vi "GraphView(Cursor).vi"() -> ()   [LabVIEW 2014]
uses:
  <vilib>/Utility/miscctls.llb/LVCursorListTypeDef.ctl
  GlobalData/GlobalData.vi
panel:
  out "クラスタ 2":T1
  out "クラスタ":T1
  in  "中央に表示A":bool
  in  "対象スケール(Y)":u16(ring) items=["回転M1１", "回転M23", "トルクM1", "トルクM23", "温度１", "温度２", "温度３", "温度４"]
  in  "削除B":bool
  in  "カーソル名称":string
  in  "カーソルB":u16(ring) items=["あ", "い"]
  in  "カーソルA":u16(ring) items=["あ", "い"]
  in  "トレース追加ボタン":bool
  in  "削除A":bool
  in  "表 2":string[][](table)
  in  "カラー":u32(colorbox)
  in  "カーソルモード":u16(ring) items=["フリー", "データ"]
  in  "対象CH":u16(ring) items=["自動", "No.", "時間HH:MM:SS.S", "M1回転rpm", "M2回転rpm", "M3回転rpm", "M1トルクN･m", "M2トルクN･m", "M3トルクN･m", "", "", "", "", "", "", "", "", "", "", "供試体温度1℃", "供試体温度2℃", "供試体温度3℃", "動力盤温度℃", "軸受温度1℃", "軸受温度2℃", "軸受温度3℃", "", "効率"]
  out "カーソルリスト":T2
  out "表":string[][](table)
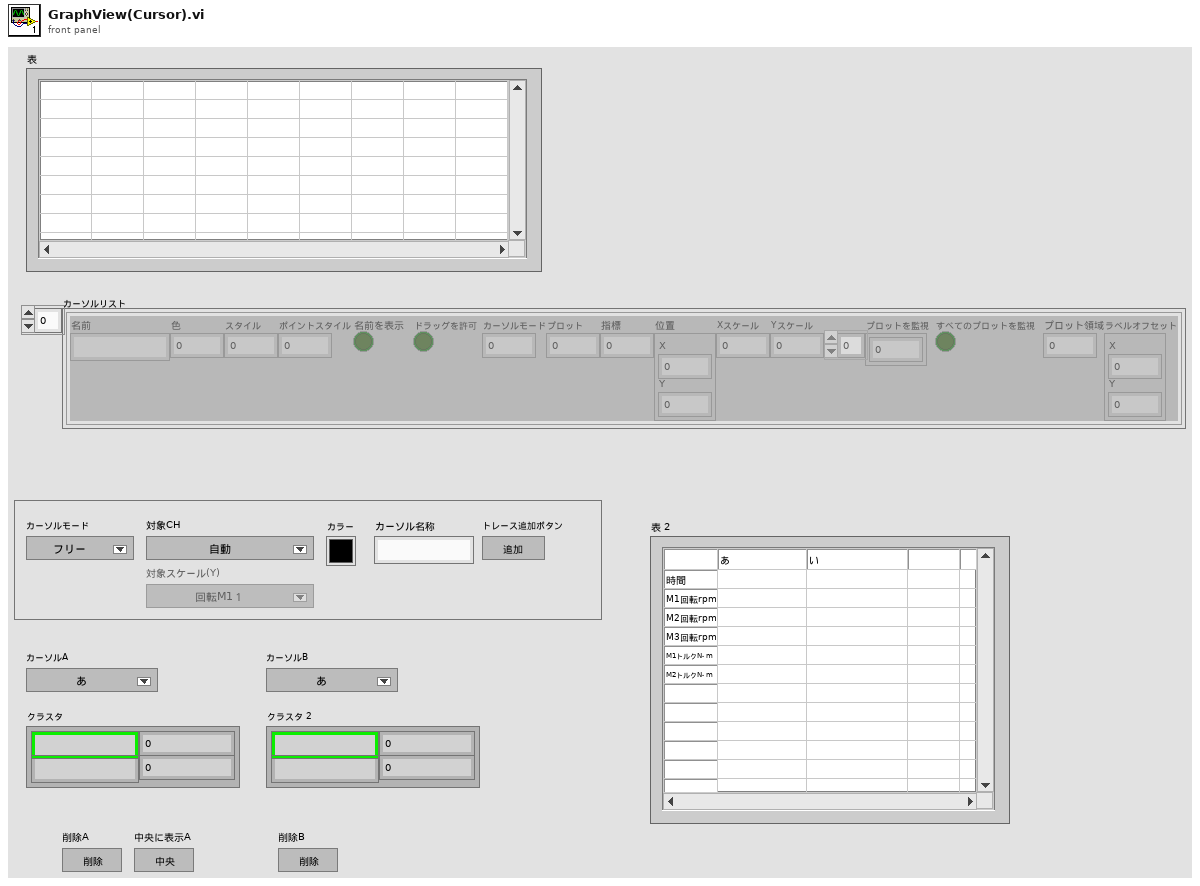
[diagram p1: front panel]
types:
  T1 = cluster{"X軸名":string, "X値":dbl, "Y軸名":string, "Y値":dbl}
  T2 = typedef "LVCursorListTypeDef.ctl" = cluster{"Name":string, "Color":u32, "Style":u8, "Point Style":u8, "Name Visible":bool, "Allow Drag":bool, "Cursor Mode":u32, "Plot":i32, "Index":i32, "Position":cluster{"X":dbl, "Y":dbl}, "X Scale":u32, "Y Scale":u32, "Watch Plots":i32[], "Watch All Plots":bool, "Plot Area":i32, "Label Offset":cluster{"X":dbl, "Y":dbl}}[]
  T3 = enum8{"Enabled", "Disabled", "Disabled and Grayed Out"}
  T4 = cluster{"Name":string, "Color":u32, "Style":u8, "Point Style":u8, "Name Visible":bool, "Allow Drag":bool, "Cursor Mode":u32, "Plot":i32, "Index":i32, "Position":cluster{"X":dbl, "Y":dbl}, "X Scale":u32, "Y Scale":u32, "Watch Plots":i32[], "Watch All Plots":bool, "Plot Area":i32, "Label Offset":cluster{"X":dbl, "Y":dbl}}
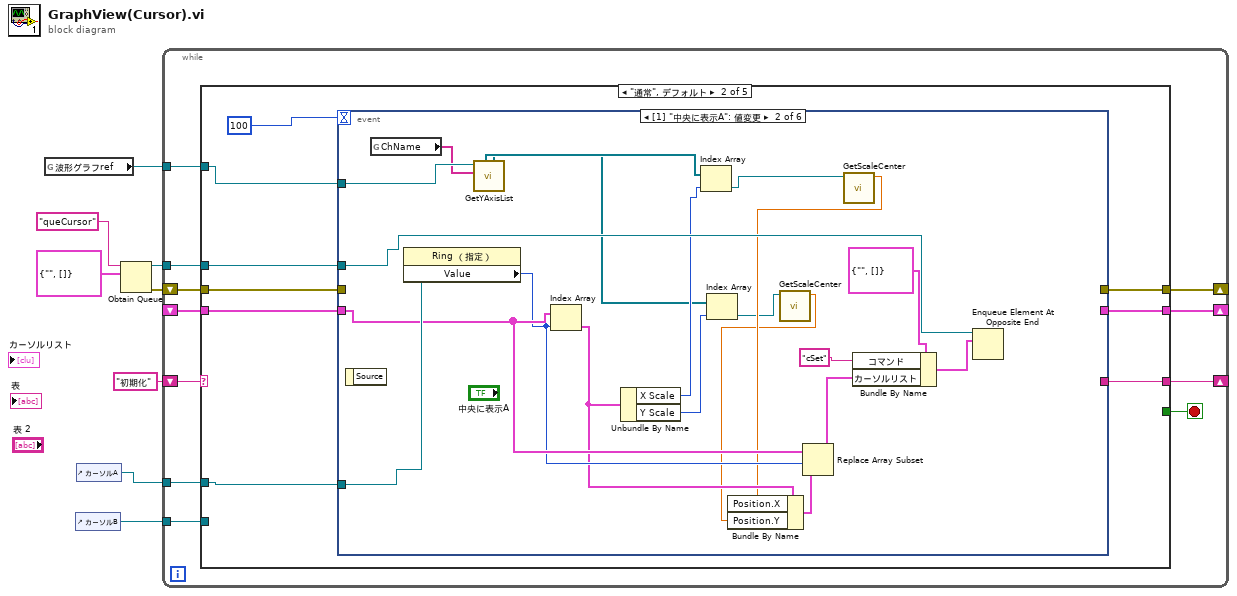
[diagram p0: block diagram]
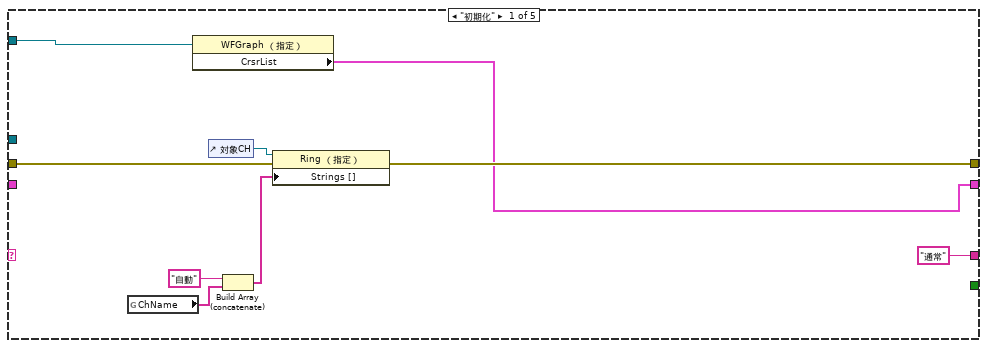
[diagram p2: hidden frame]
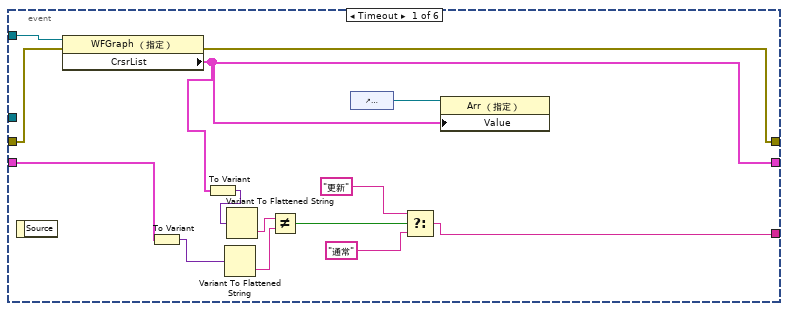
[diagram p3: hidden frame]
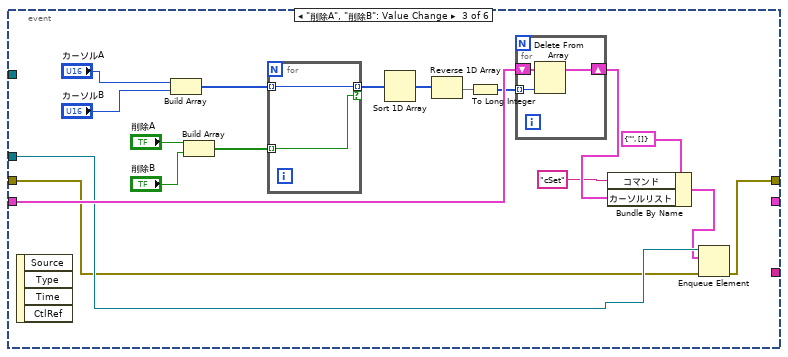
[diagram p4: hidden frame]
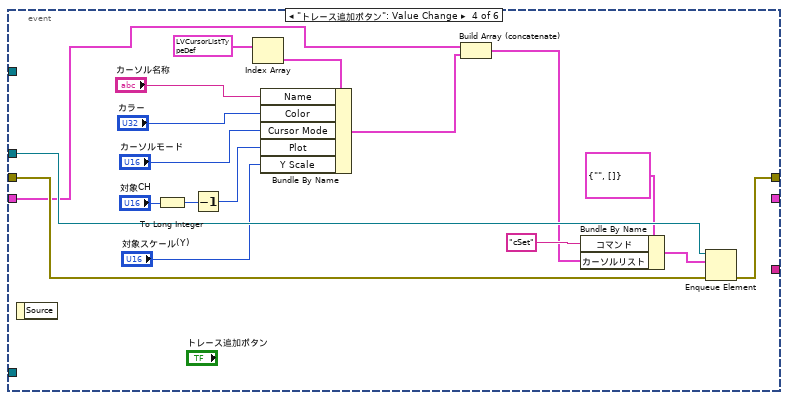
[diagram p5: hidden frame]
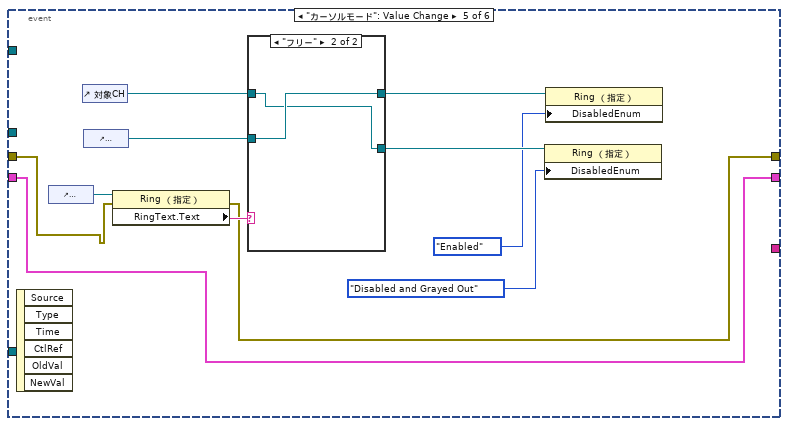
[diagram p6: hidden frame]
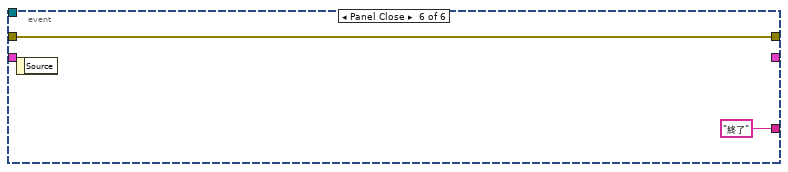
[diagram p8: hidden frame]
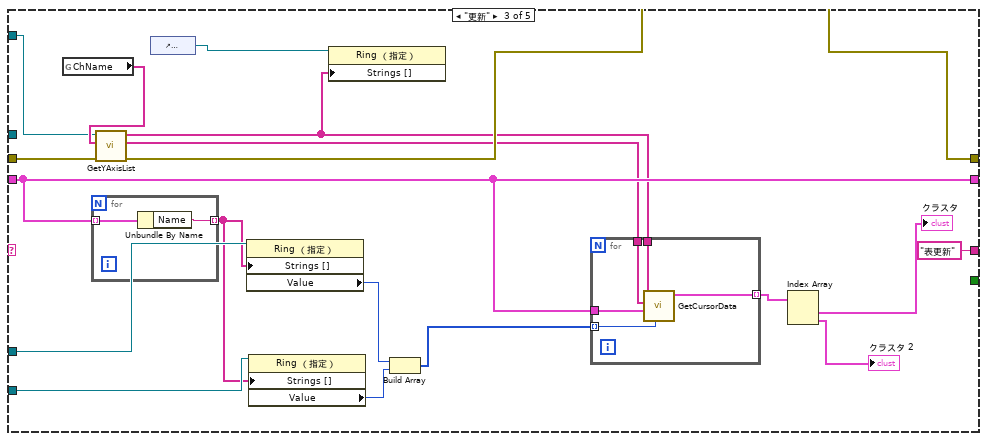
[diagram p9: hidden frame]
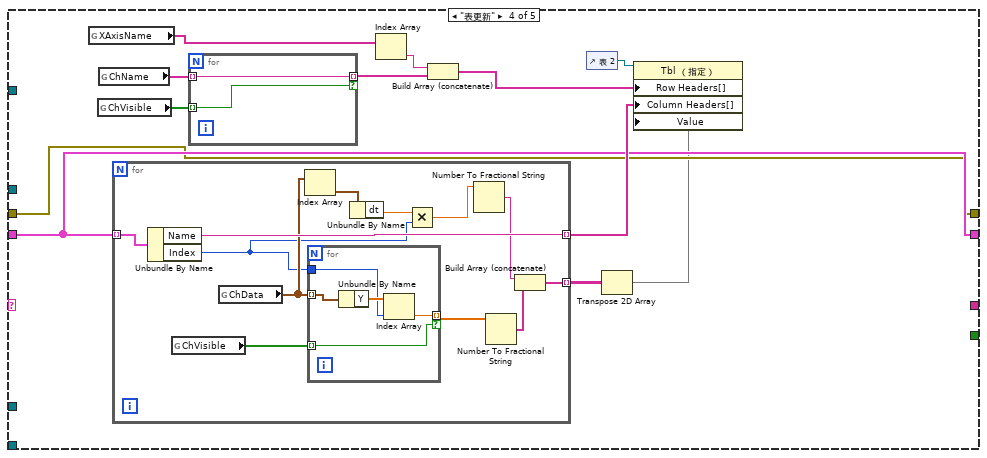
[diagram p10: hidden frame]
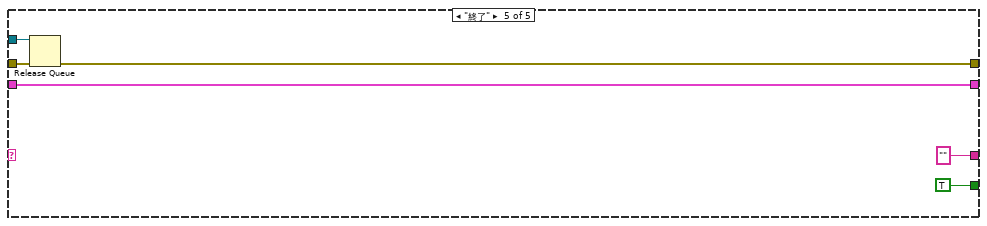
[diagram p11: hidden frame]
diagram:
  n1 = global read "GlobalData.vi" "波形グラフref"() -> (w3:refnum<vi>)
  n2 = control-ref of="カーソルB"() -> (w1:refnum<vi>)
  n3 = control-ref of="カーソルA"() -> (w2:refnum<vi>)
  n4 = Obtain Queue(name (unnamed)="queCursor" ("名前（名前なし）"), element data type=cluster{"コマンド":string, "カーソルリスト":T2} {"コマンド"="", "カーソルリスト"=[]}) -> (queue out=w4:refnum<queue>, error out=w7:errorcluster)  [unwired: 3 in, 1 out]
  n5 = while {
    tunnel: w4 -> [w17]
    shift-right: [w16] -> _
    shift-left: w7 -> [w18]
    shift-right: [w14] -> _
    shift-left: "初期化" -> [w15]
    shift-right: [w13] -> _
    shift-left: _ -> [w12]
    tunnel: w3 -> [w11]
    tunnel: w2 -> [w10]
    tunnel: w1 -> [w9]
    stop <- w19 stop-if-true
    n6 = case shown="\"通常\", デフォルト" w15 {
      tunnel: [_ _ _ _ TRUE] -> w19
      tunnel: w18 -> [w27 w37 w145 w156 w189]
      tunnel: w17 -> [_ w35 _ _ w187]
      tunnel: [w26 w34 w144 w156 w188] -> w16
      tunnel: ["通常" w33 "表更新" _ ""] -> w14
      tunnel: [w20 w32 w147 w157 w186] -> w13
      tunnel: w12 -> [_ w31 w147 w157 w186]
      tunnel: w11 -> [w21 w30 w139 _ _]
      tunnel: w10 -> [_ w29 w146 _ _]
      tunnel: w9 -> [_ _ w138 _ _]
      frame "初期化" {
        n7 = global read "GlobalData.vi" "ChName"() -> (w23:string[])
        n8 = property class="WFGraph （指定）"(reference=w21) -> ("CrsrList"=w20:T2)  [unwired: 1 in, 2 out]
        n9 = control-ref of="対象CH"() -> (w25:refnum<vi>)
        n10 = Build Array (concatenate)("自動", w23) -> (w22:string[])
        n11 = property class="Ring （指定）"(reference=w25, error in=w27, "Strings []"=w22) -> (error out=w26:errorcluster)  [unwired: 1 out]
      }
      frame "通常", Default {
        n12 = event shown="[1] \"中央に表示A\": 値変更" {
          selector: _ -> [_ _ _ _ _ _]
          dyn-events: _ -> [_ _ _ _ _ _]
          timeout: 100 -> [_ _ _ _ _ _]
          tunnel: w37 -> [w49 _ w73 w108 w115 w129]
          tunnel: w35 -> [_ w70 w78 w112 _ _]
          tunnel: [w48 _ w72 w107 w114 w129] -> w34
          tunnel: [w38 _ _ _ _ "終了"] -> w33
          tunnel: [w42 _ _ _ w113 _] -> w32
          tunnel: w31 -> [w46 w60 w81 w97 w113 _]
          tunnel: w30 -> [w50 w67 _ _ _ _]
          tunnel: w29 -> [_ w71 _ _ _ _]
          event Timeout {
            n13 = event-data() -> ()  [unwired: 1 in, 1 out]
            n14 = property class="WFGraph （指定）"(reference=w50, error in=w49) -> (error out=w48:errorcluster, "CrsrList"=w42:T2)  [unwired: 1 out]
            n15 = To Variant(anything=w46) -> (Variant=w45:variant)
            n16 = To Variant(anything=w42) -> (Variant=w47:variant)
            n17 = Variant To Flattened String(Variant=w45) -> (data string=w43:string)  [unwired: 1 out]
            n18 = Variant To Flattened String(Variant=w47) -> (data string=w44:string)  [unwired: 1 out]
            n19 = Not Equal?(x=w44, y=w43) -> (x != y?=w41:bool)
            n20 = control-ref of="カーソルリスト"() -> (w51:refnum<vi>)
            n21 = Select(t="更新", s=w41, f="通常") -> (s? t:f=w38:string)
            n22 = property class="Arr （指定）"(reference=w51, "Value"=w42) -> ()  [unwired: 1 in, 2 out]
          }
          event "中央に表示A": Value Change {
            n23 = event-data() -> ()  [unwired: 1 in, 1 out]
            n24 = global read "GlobalData.vi" "ChName"() -> (w66:string[])
            n25 = property class="Ring （指定）"(reference=w71) -> ("Value"=w59:u16)  [unwired: 1 in, 2 out]
            n26 = call "GetYAxisList.vi"("ChName[]"=w66, "波形グラフref"=w67) -> ("Y軸ref[]"=w63:refnum<vi>[], "X軸ref[]"=w65:refnum<vi>[])  [unwired: 4 in, 4 out]
            n27 = Index Array(array=w60, index=w59) -> (element=w58:T4)
            n28 = Unbundle By Name(w58) -> ("X Scale"=w64:u32, "Y Scale"=w62:u32)
            n29 = Index Array(array=w65, index=w64) -> (element=w57:refnum<vi>)
            n30 = Index Array(array=w63, index=w62) -> (element=w55:refnum<vi>)
            n31 = call "GetScaleCenter.vi"("GraphScale入力"=w55) -> ("数値"=w54:dbl)  [unwired: 10 in]
            n32 = call "GetScaleCenter.vi"("GraphScale入力"=w57) -> ("数値"=w56:dbl)  [unwired: 10 in]
            n33 = Bundle By Name(cluster=w58, "Position.X"=w56, "Position.Y"=w54) -> (w53:T4)
            n34 = Replace Array Subset(array=w60, new element=w53, index=w59) -> (w61:T2)
            n35 = Bundle By Name(cluster=cluster{"コマンド":string, "カーソルリスト":T2} {"コマンド"="", "カーソルリスト"=[]}, "コマンド"="cSet", "カーソルリスト"=w61) -> (w52:cluster{"コマンド":string, "カーソルリスト":T2})
            n36 = Enqueue Element At Opposite End(queue=w70, element=w52) -> ()  [unwired: 2 in, 3 out]
          }
          event "削除A", "削除B": Value Change {
            n37 = event-data() -> ()  [unwired: 1 in, 4 out]
            n38 = Build Array("カーソルA", "カーソルB") -> (w85:u16[])
            n39 = Build Array("削除A", "削除B") -> (w84:bool[])
            n40 = for {
              tunnel: w85 -> [w94] mode=indexing
              tunnel: w84 -> [w93] mode=indexing
              tunnel: [w94] -> w83 mode=indexing if=w93
            }
            n41 = Sort 1D Array(array=w83) -> (sorted array=w82:u16[])
            n42 = Reverse 1D Array(array=w82) -> (reversed array=w80:u16[])
            n43 = To Long Integer(number=w80) -> (32bit integer=w79:i32[])
            n44 = for {
              tunnel: w79 -> [w91] mode=indexing
              shift-right: [w90] -> w76
              shift-left: w81 -> [w92]
              n45 = Delete From Array(array=w92, index=w91) -> (array with subset deleted=w90:T2)  [unwired: 1 in, 1 out]
            }
            n46 = Bundle By Name(cluster=cluster{"コマンド":string, "カーソルリスト":T2} {"コマンド"="", "カーソルリスト"=[]} ("要素"), "コマンド"="cSet", "カーソルリスト"=w76) -> (w74:cluster{"コマンド":string, "カーソルリスト":T2})
            n47 = Enqueue Element(queue=w78, element=w74, error in (no error)=w73) -> (error out=w72:errorcluster)  [unwired: 1 in, 2 out]
          }
          event "トレース追加ボタン": Value Change {
            n48 = event-data() -> ()  [unwired: 1 in, 1 out]
            n49 = To Long Integer(number="対象CH") -> (32bit integer=w99:i32)
            n50 = Decrement(x=w99) -> (x-1=w98:i32)
            n51 = Index Array(array=T2 [{"Name"="", "Color"=16776960, "Style"=8, "Point Style"=13, "Name Visible"=FALSE, "Allow Drag"=TRUE, "Cursor Mode"=1, "Plot"=-1, "Index"=4, "Position"={"X"=0.4, "Y"=3866.003327}, "X Scale"=0, "Y Scale"=3, "Watch Plots"=[], "Watch All Plots"=FALSE, "Plot Area"=0, "Label Offset"={"X"=0.0007092198581559739, "Y"=84.63280531552164}}] ("カーソルリスト")) -> (element=w106:T4)  [unwired: 1 in]
            n52 = Bundle By Name(cluster=w106, "Name"="カーソル名称", "Color"="カラー", "Cursor Mode"="カーソルモード", "Plot"=w98, "Y Scale"="対象スケール(Y)") -> (w105:T4)
            n53 = Build Array (concatenate)(w97, w105) -> (w104:T2)
            n54 = Bundle By Name(cluster=cluster{"コマンド":string, "カーソルリスト":T2} {"コマンド"="", "カーソルリスト"=[]}, "コマンド"="cSet", "カーソルリスト"=w104) -> (w109:cluster{"コマンド":string, "カーソルリスト":T2})
            n55 = Enqueue Element(queue=w112, element=w109, error in (no error)=w108) -> (error out=w107:errorcluster)  [unwired: 1 in, 2 out]
          }
          event "カーソルモード": Value Change {
            n56 = event-data() -> ()  [unwired: 1 in, 6 out]
            n57 = control-ref of="カーソルモード"() -> (w121:refnum<vi>)
            n58 = control-ref of="対象CH"() -> (w123:refnum<vi>)
            n59 = control-ref of="対象スケール(Y)"() -> (w122:refnum<vi>)
            n60 = property class="Ring （指定）"(reference=w121, error in=w115) -> (error out=w114:errorcluster, "RingText.Text"=w120:string)  [unwired: 1 out]
            n61 = case shown="\"フリー\"" w120 {
              tunnel: w123 -> [w125 w126]
              tunnel: w122 -> [w124 w127]
              tunnel: [w125 w127] -> w119
              tunnel: [w124 w126] -> w118
              frame "データ", Default {
              }
              frame "フリー" {
              }
            }
            n62 = property class="Ring （指定）"(reference=w118, "DisabledEnum"=T3."Disabled and Grayed Out" ("無効")) -> ()  [unwired: 1 in, 2 out]
            n63 = property class="Ring （指定）"(reference=w119, "DisabledEnum"=T3."Enabled" ("無効")) -> ()  [unwired: 1 in, 2 out]
          }
          event Panel Close {
            n64 = event-data() -> ()  [unwired: 1 in, 1 out]
          }
        }
      }
      frame "更新" {
        n65 = global read "GlobalData.vi" "ChName"() -> (w140:string[])
        n66 = for {
          tunnel: w147 -> [w154] mode=indexing
          tunnel: [w153] -> w137 mode=indexing
          n67 = Unbundle By Name(w154) -> ("Name"=w153:string)
        }
        n68 = call "GetYAxisList.vi"("error in (no error)"=w145, "ChName[]"=w140, "波形グラフref"=w139) -> ("error out"=w144:errorcluster, "X軸名称[]"=w142:string[], "Y軸名称[]"=w141:string[])  [unwired: 3 in, 3 out]
        n69 = control-ref of="対象スケール(Y)"() -> (w143:refnum<vi>)
        n70 = property class="Ring （指定）"(reference=w146, "Strings []"=w137) -> ("Value"=w136:u16)  [unwired: 1 in, 2 out]
        n71 = property class="Ring （指定）"(reference=w138, "Strings []"=w137) -> ("Value"=w135:u16)  [unwired: 1 in, 2 out]
        n72 = property class="Ring （指定）"(reference=w143, "Strings []"=w141) -> ()  [unwired: 1 in, 2 out]
        n73 = Build Array(w136, w135) -> (w134:u16[])
        n74 = for {
          tunnel: w147 -> [w152]
          tunnel: [w151] -> w133 mode=indexing
          tunnel: w142 -> [w150]
          tunnel: w141 -> [w149]
          tunnel: w134 -> [w148] mode=indexing
          n75 = call "GetCursorData.vi"("Value"=w148, "CrsrList"=w152, "X軸名称[]"=w150, "Y軸名称[]"=w149) -> ("カーソルデータ"=w151:T1)  [unwired: 6 in, 1 out]
        }
        n76 = Index Array(array=w133) -> (element #1=→"クラスタ":T1, element #2=→"クラスタ 2":T1)  [unwired: 2 in]
      }
      frame "表更新" {
        n77 = global read "GlobalData.vi" "XAxisName"() -> (w164:string[])
        n78 = global read "GlobalData.vi" "ChVisible"() -> (w165:bool[])
        n79 = global read "GlobalData.vi" "ChName"() -> (w166:string[])
        n80 = for {
          tunnel: w157 -> [w180] mode=indexing
          tunnel: [w179] -> w159 mode=indexing
          tunnel: [w172] -> w158 mode=indexing
          n81 = Unbundle By Name(w180) -> ("Name"=w179:string, "Index"=w175:i32)
          n82 = global read "GlobalData.vi" "ChVisible"() -> (w171:bool[])
          n83 = global read "GlobalData.vi" "ChData"() -> (w178:waveform(dbl)[])
          n84 = Index Array(array=w178) -> (element=w177:waveform(dbl))  [unwired: 1 in]
          n85 = for {
            tunnel: w175 -> [w183]
            tunnel: w178 -> [w185] mode=indexing
            tunnel: [w182] -> w173 mode=indexing if=w181
            tunnel: w171 -> [w181] mode=indexing
            n86 = Unbundle By Name(w185) -> ("Y"=w184:dbl[])
            n87 = Index Array(array=w184, index=w183) -> (element=w182:dbl)
          }
          n88 = Unbundle By Name(w177) -> ("dt"=w176:dbl)
          n89 = Multiply(x=w176, y=w175) -> (x*y=w170:dbl)
          n90 = Number To Fractional String(number=w170) -> (F-format string=w169:string)  [unwired: 3 in]
          n91 = Number To Fractional String(number=w173) -> (F-format string=w174:string[])  [unwired: 3 in]
          n92 = Build Array (concatenate)(w169, w174) -> (w172:string[])
        }
        n93 = for {
          tunnel: w166 -> [w168] mode=indexing
          tunnel: [w168] -> w162 mode=indexing if=w167
          tunnel: w165 -> [w167] mode=indexing
        }
        n94 = Index Array(array=w164) -> (element=w163:string)  [unwired: 1 in]
        n95 = Build Array (concatenate)(w163, w162) -> (w160:string[])
        n96 = control-ref of="表 2"() -> (w161:refnum<vi>)
        n97 = Transpose 2D Array(2D array=w158) -> (transposed array=w155:string[][])
        n98 = property class="Tbl （指定）"(reference=w161, "Row Headers[]"=w160, "Column Headers[]"=w159, "Value"=w155) -> ()  [unwired: 1 in, 2 out]
      }
      frame "終了" {
        n99 = Release Queue(queue=w187, error in (no error)=w189) -> (error out=w188:errorcluster)  [unwired: 1 in, 2 out]
      }
    }
  }
